vi "enable disable test.vi"() -> ()   [LabVIEW 2019]
panel:
  in  "Numeric":dbl=10.0
  out "String 2":string
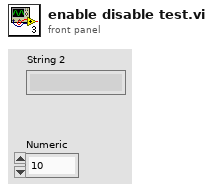
[diagram p1: front panel]
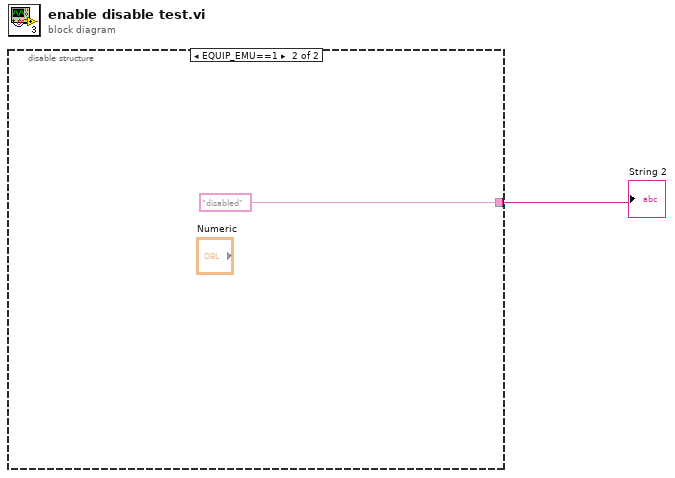
[diagram p0: block diagram]
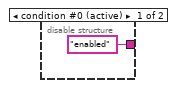
[diagram p2: hidden frame]
diagram:
  n1 = disable-structure shown="EQUIP_EMU==1" {
    disable-tunnel: ["enabled" ("String 2") "disabled" ("String 2")] -> w1
    frame condition #0 (active) {
    }
    frame condition #1 {
    }
  }
  "String 2" <- w1
